vi "ABCtoDQ_2PhaseUnitaryMagnitude_src.vi"(0 "A":sgl, 5 "B":sgl, 9 "Theta":sgl) -> (4 "direct":sgl, 6 "quadrature":sgl, 8 "alpha":sgl, 10 "beta":sgl, 13 "sinx":sgl, 14 "cosx":sgl)   [LabVIEW 2015]
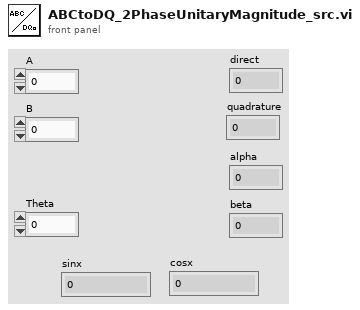
[diagram p1: front panel]
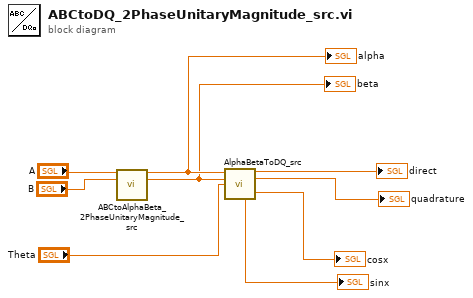
[diagram p0: block diagram]
diagram:
  n1 = call "ABCtoAlphaBeta_2PhaseUnitaryMagnitude_src.vi"("A"="A", "B"="B") -> ("alpha"=w4:sgl, "beta"=w3:sgl)  [unwired: 12 in]
  "alpha" <- w4
  "beta" <- w3
  n2 = call "AlphaBetaToDQ_src.vi"("alpha"=w4, "beta"=w3, "theta"="Theta") -> ("direct"=→"direct":sgl, "quadrature"=→"quadrature":sgl, "sinx"=→"sinx":sgl, "cosx"=→"cosx":sgl)  [unwired: 9 in]
